vi "Load Products.vi"(8 "error in (no error)":errorcluster, 11 "English Picker in":refnum<class "English Picker.lvclass">) -> (0 "error out":errorcluster, 3 "English Picker out":refnum<class "English Picker.lvclass">)   [LabVIEW 2020, in "English Picker.lvlib" / "English Picker.lvclass"]
uses:
  English Picker.lvclass
  D:/Storage/Source Code/Clase AF/ClaseAF/05 AF Camera/Products Picker/Products Picker.lvclass
  Products Picker/Products Picker.lvclass/Products Picker.ctl
  Products Picker/Products Picker.lvclass
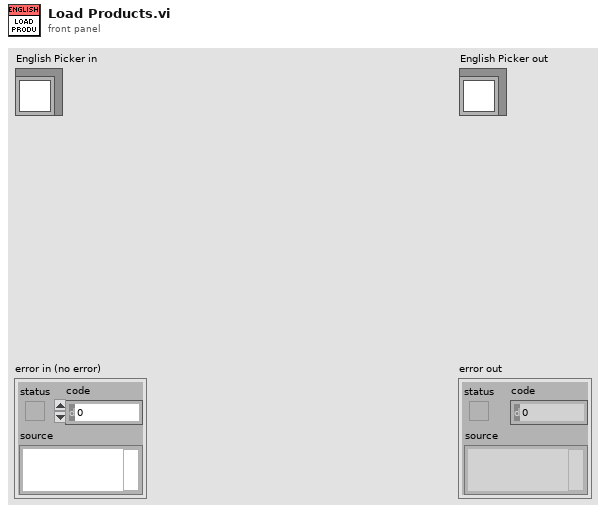
[diagram p1: front panel]
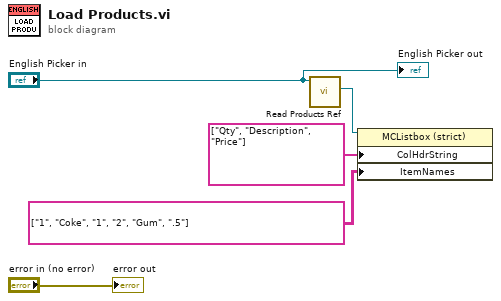
[diagram p0: block diagram]
diagram:
  n1 = call "Read Products Ref.vi"("Products Picker in"="English Picker in") -> ("Products Ref"=w2:refnum<vi>)  [unwired: 9 in, 1 out]
  n2 = property class="MCListbox (strict)"(reference=w2, "ColHdrString"=string[] ["Qty", "Description", "Price"] ("Column Header Strings[]"), "ItemNames"=string[][] [["1", "Coke", "1"], ["2", "Gum", ".5"]] ("Item Names")) -> ()  [unwired: 1 in, 2 out]
  "error out" <- "error in (no error)"
  "English Picker out" <- "English Picker in"
